vi "comparing result.vi"() -> ()   [LabVIEW 2020]
uses:
  common/record_file_handler/VFH-VNA_File_Handler.lvlib
panel:
  out "size(s)":i32
  in  "Checkbox":bool
  out "Data Points":i32
  out "Cluster":T1 {"Z''" format="%#_5p"; "Z'" format="%#_5p"; "|Z|" format="%#_5p"; "Loss" format="%#_5p"; "Deg" format="%#_5p"; "Phi" format="%#_5p"; "Mag" format="%#_5p"; "S11 I" format="%#_5p"; "S11 R" format="%#_5p"}
  out "Array":dbl[](array[numeric]) format="%#_5p"
  out "Freq":dbl format="%#_6p"
  in  "index":i32
  in  "Stop":bool
  in  "Folder Path":path=path "C:/NanoVNA-App/Recordings/2024-07-26 09-29-22"
  in  "Tab Control":enum32{"Page 1", "Page 2"}(tab)
  out "Complex":cluster{"Frequency":dbl[], "S21_Imag":dbl[]}[](graph)
  in  "Log Raw":bool
  out "Calc":cluster{"Frequency":dbl[], "S11_Imag":dbl[]}[](graph)
  out "Raw":cluster{"Frequency":dbl[], "S21_Imag":dbl[]}[](graph)
  in  "Log calc":bool
  in  "Log complex":bool
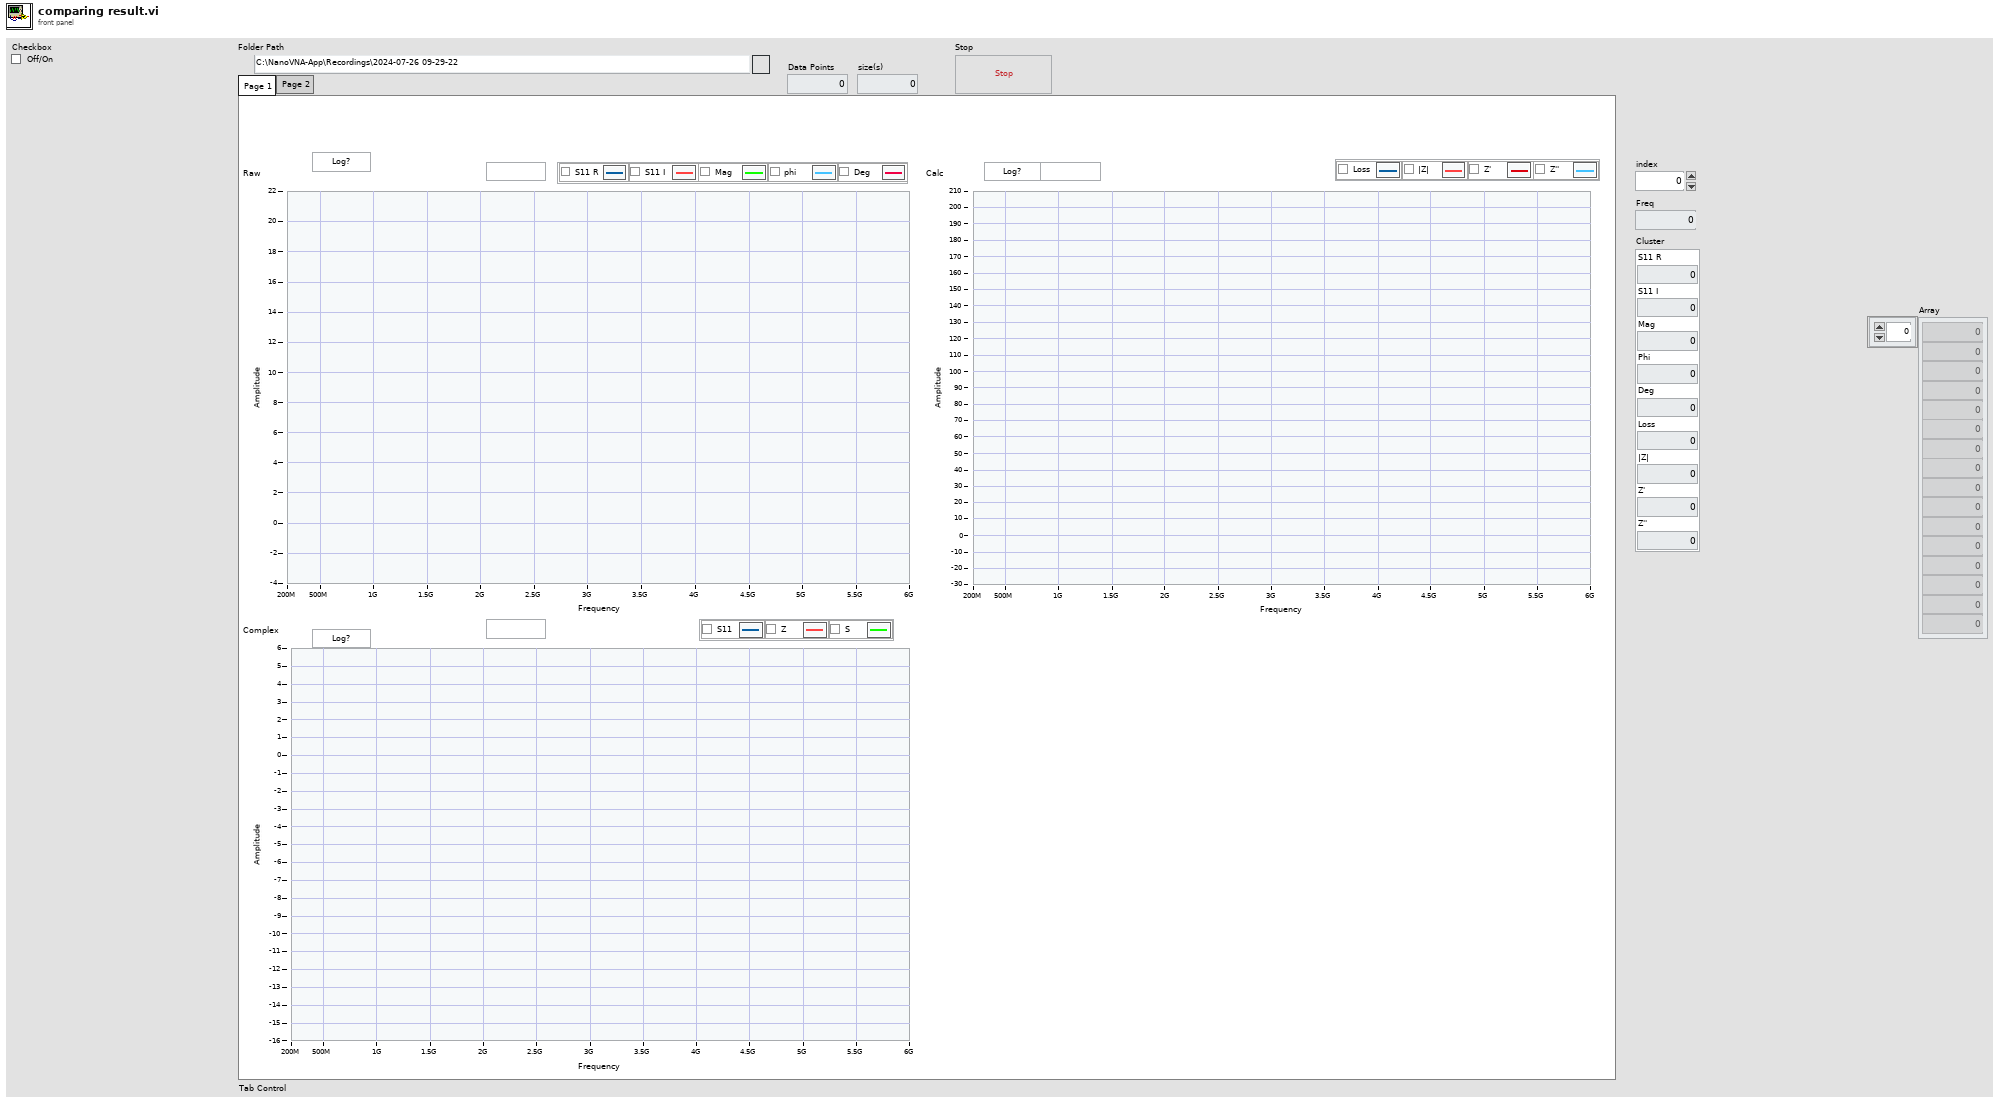
[diagram p1: front panel]
types:
  T1 = cluster{"S11 R":dbl, "S11 I":dbl, "Mag":dbl, "Phi":dbl, "Deg":dbl, "Loss":dbl, "|Z|":dbl, "Z'":dbl, "Z''":dbl}
  T2 = typedef "VFH-VNA_File_Handler.lvlib/VFH-file_cluster-LabVIEWVNA.ctl" = cluster{"Frequency":dbl[], "S1_Real":dbl[], "S1_Imag":dbl[], "S11_Real":dbl[], "S11_Imag":dbl[], "S21_Real":dbl[], "S21_Imag":dbl[]}
  T3 = typedef "VFH-VNA_File_Handler.lvlib/VFH-file_cluster-NanoVNA.ctl" = cluster{"Frequency":dbl[], "S11_Real":dbl[], "S11_Imag":dbl[], "S21_Real":dbl[], "S21_Imag":dbl[], "S12_Real":dbl[], "S12_Imag":dbl[], "S22_Real":dbl[], "S22_Imag":dbl[]}
  T4 = cluster{"Complex Input":cluster{"Frequency":dbl[], "Array":cdb[]}, "Complex Z":cluster{"Frequency":dbl[], "Array":cdb[]}, "Complex S":cluster{"Frequency":dbl[], "Array":cdb[]}}
  T5 = cluster{"Loss":cluster{"Frequency":dbl[], "Array":dbl[]}, "Z Modulus":cluster{"Frequency":dbl[], "Array":dbl[]}, "Z'":cluster{"Frequency":dbl[], "Array":dbl[]}, "Z''":cluster{"Frequency":dbl[], "Array":dbl[]}}
  T6 = cluster{"S11'":cluster{"Frequency":dbl[], "S11_Real":dbl[]}, "S11''":cluster{"Frequency":dbl[], "S11_Real":dbl[]}, "Magnitude":cluster{"Frequency":dbl[], "Array":dbl[]}, "Eta":cluster{"Frequency":dbl[], "Array":dbl[]}, "Phase":cluster{"Frequency":dbl[], "Array":dbl[]}}
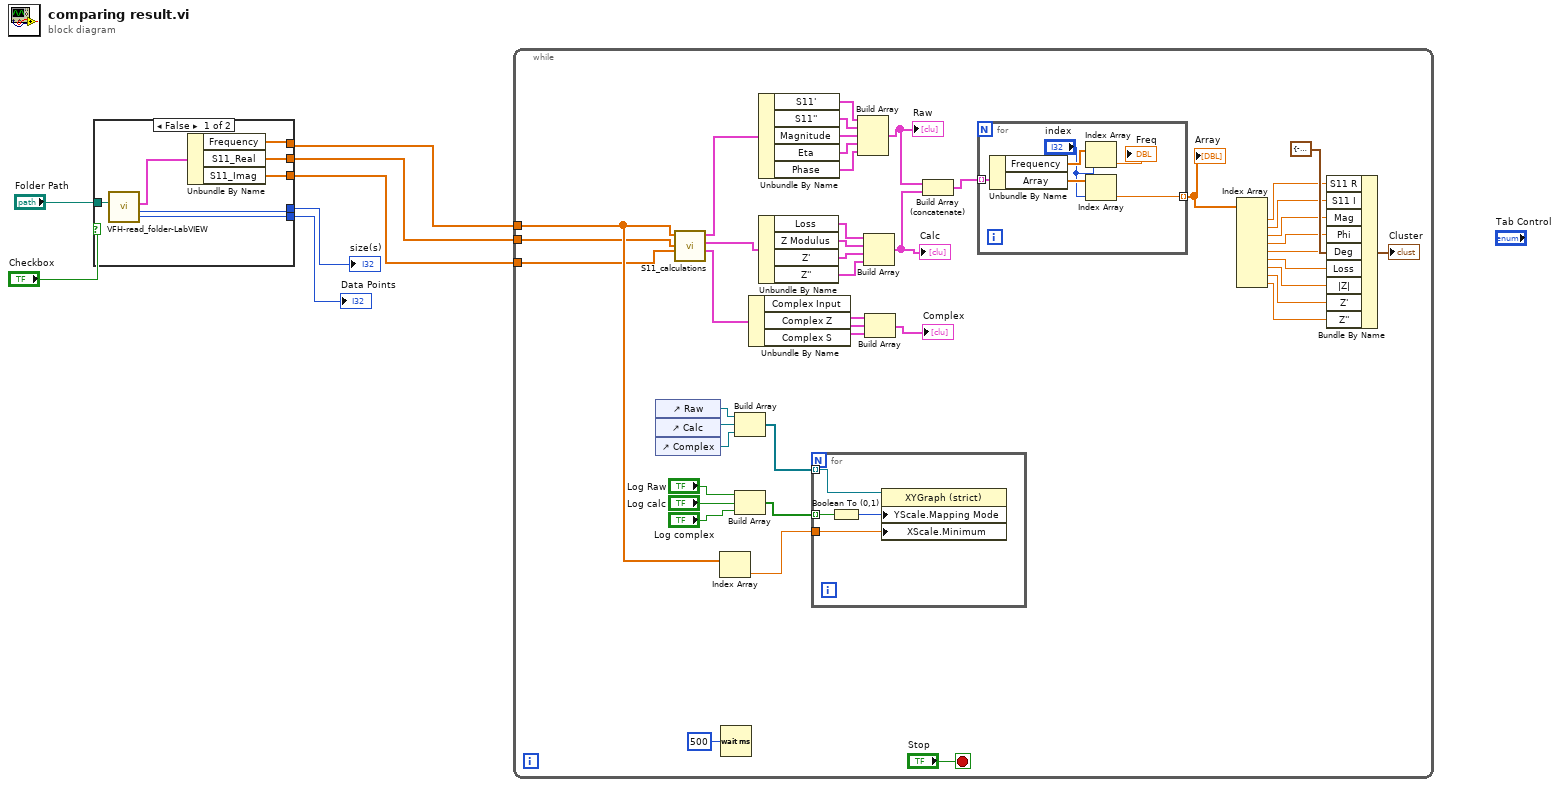
[diagram p0: block diagram]
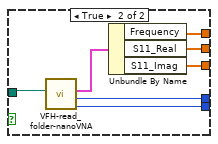
[diagram p2: hidden frame]
diagram:
  n1 = case shown="False" "Checkbox" {
    tunnel: "Folder Path" -> [w14 w21]
    tunnel: [w9 w20] -> w6
    tunnel: [w8 w19] -> w5
    tunnel: [w12 w17] -> w3
    tunnel: [w11 w16] -> w2
    tunnel: [w10 w15] -> w1
    frame False {
      n2 = call "VFH-read_folder-LabVIEW.vi"("Folder Path"=w14) -> ("Samples"=w8:i32, "size(s)"=w9:i32, "avg output"=w13:T2)  [unwired: 8 in]
      n3 = Unbundle By Name(w13) -> ("Frequency"=w12:dbl[], "S11_Real"=w11:dbl[], "S11_Imag"=w10:dbl[])
    }
    frame True {
      n4 = call "VFH-read_folder-nanoVNA.vi"("Folder Path"=w21) -> ("Data Points"=w19:i32, "size(s)"=w20:i32, "avg output"=w18:T3)  [unwired: 8 in]
      n5 = Unbundle By Name(w18) -> ("Frequency"=w17:dbl[], "S11_Real"=w16:dbl[], "S11_Imag"=w15:dbl[])
    }
  }
  "size(s)" <- w6
  "Data Points" <- w5
  n6 = while {
    tunnel: w3 -> [w24]
    tunnel: w2 -> [w23]
    tunnel: w1 -> [w22]
    stop <- "Stop" stop-if-true
    n7 = control-ref of="Raw"() -> (w33:refnum<vi>)
    n8 = control-ref of="Calc"() -> (w32:refnum<vi>)
    n9 = control-ref of="Complex"() -> (w31:refnum<vi>)
    n10 = call "S11_calculations.vi"("S11_Imag"=w22, "S11_Real"=w23, "Frequency"=w24) -> ("Complex"=w50:T4, "Calc"=w60:T5, "Raw"=w66:T6)  [unwired: 6 in]
    n11 = Index Array(array=w24) -> (element=w25:dbl)  [unwired: 1 in]
    n12 = Wait (ms)(milliseconds to wait=u32 500) -> ()  [unwired: 1 out]
    n13 = Build Array(w33, w32, w31) -> (w30:refnum<vi>[])
    n14 = Build Array("Log Raw", "Log calc", "Log complex") -> (w26:bool[])
    n15 = Unbundle By Name(w50) -> ("Complex Input"=w51:cluster{"Frequency":dbl[], "Array":cdb[]}, "Complex Z"=w52:cluster{"Frequency":dbl[], "Array":cdb[]}, "Complex S"=w53:cluster{"Frequency":dbl[], "Array":cdb[]})
    n16 = Unbundle By Name(w66) -> ("S11'"=w65:cluster{"Frequency":dbl[], "S11_Real":dbl[]}, "S11''"=w64:cluster{"Frequency":dbl[], "S11_Real":dbl[]}, "Magnitude"=w63:cluster{"Frequency":dbl[], "Array":dbl[]}, "Eta"=w62:cluster{"Frequency":dbl[], "Array":dbl[]}, "Phase"=w61:cluster{"Frequency":dbl[], "Array":dbl[]})
    n17 = Unbundle By Name(w60) -> ("Loss"=w59:cluster{"Frequency":dbl[], "Array":dbl[]}, "Z Modulus"=w58:cluster{"Frequency":dbl[], "Array":dbl[]}, "Z'"=w57:cluster{"Frequency":dbl[], "Array":dbl[]}, "Z''"=w56:cluster{"Frequency":dbl[], "Array":dbl[]})
    n18 = for {
      tunnel: w30 -> [w70] mode=indexing
      tunnel: w26 -> [w69] mode=indexing
      tunnel: w25 -> [w67]
      n19 = Boolean To (0,1)(Boolean=w69) -> (0, 1=w68:i16)
      n20 = property class="XYGraph (strict)"(reference=w70, "YScale.Mapping Mode"=w68, "XScale.Minimum"=w67) -> ()  [unwired: 1 in, 2 out]
    }
    n21 = Build Array(w65, w64, w63, w62, w61) -> (w47:cluster{"Frequency":dbl[], "Array":dbl[]}[])
    "Raw" <- w47
    n22 = Build Array(w59, w58, w57, w56) -> (w48:cluster{"Frequency":dbl[], "Array":dbl[]}[])
    "Calc" <- w48
    n23 = Build Array(w51, w52, w53) -> (→"Complex":cluster{"Frequency":dbl[], "Array":cdb[]}[])
    n24 = Build Array (concatenate)(w47, w48) -> (w46:cluster{"Frequency":dbl[], "Array":dbl[]}[])
    n25 = for {
      tunnel: w46 -> [w76] mode=indexing
      tunnel: [w71] -> w45 mode=indexing
      n26 = Unbundle By Name(w76) -> ("Frequency"=w74:dbl[], "Array"=w75:dbl[])
      n27 = Index Array(array=w74, index="index") -> (element=→"Freq":dbl)
      n28 = Index Array(array=w75, index="index") -> (element=w71:dbl)
    }
    "Array" <- w45
    n29 = Index Array(array=w45) -> (element #1=w42:dbl, element #2=w41:dbl, element #3=w40:dbl, element #4=w39:dbl, element #5=w38:dbl, element #6=w37:dbl, element #7=w36:dbl, element #8=w35:dbl, element #9=w34:dbl)  [unwired: 9 in]
    n30 = Bundle By Name(cluster=T1 {"S11 R"=-0.13079270605384616, "S11 I"=-0.13079270605384616, "Mag"=-0.13079270605384616, "Phi"=-0.13079270605384616, "Deg"=-0.13079270605384616, "Loss"=-0.13079270605384616, "|Z|"=-0.13079270605384616, "Z'"=-0.13079270605384616, "Z''"=-0.13079270605384616} ("Cluster"), "S11 R"=w42, "S11 I"=w41, "Mag"=w40, "Phi"=w39, "Deg"=w38, "Loss"=w37, "|Z|"=w36, "Z'"=w35, "Z''"=w34) -> (→"Cluster":T1)
  }
